vi "Platinum - Convert Kelvin to mV.vi"(7 "Platinum K":dbl format="%.4f") -> (8 "Platinum mV":dbl format="%.4f")   [LabVIEW 2011]
panel:
  # "PLATINUM SENSOR"
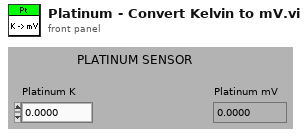
[diagram p1: front panel]
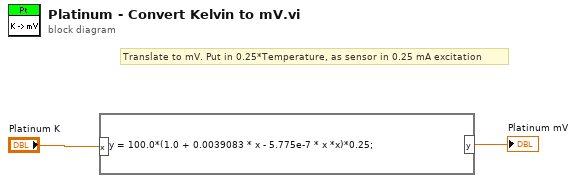
[diagram p0: block diagram]
diagram:
  # "Translate to mV. Put in 0.25*Temperature, as sensor in 0.25 mA excitation"
  n1 = formula code="y = 100.0*(1.0 + 0.0039083 * x - 5.775e-7 * x *x)*0.25;"("x"="Platinum K") -> ("y"=→"Platinum mV":dbl)
